vi "AdaptToInputs.vi"(0 "XRef":T14, 1 "Term Types":T11, 2 "State In":T1) -> (14 "Reply":T9, 15 "Fatal Error Out":T8, 16 "State Out":T1)   [LabVIEW 2020, in "Parallel Diagram Block.xnode"]
uses:
  Parallel Diagram Block.xnode
  <vilib>/XNodeSupport/XNodeXNodeRef.ctl
  <vilib>/XNodeSupport/XNodeTermTypeIDPairs.ctl
  <vilib>/XNodeSupport/XNodeTermTypeIDPair.ctl
  <vilib>/XNodeSupport/XNodeType.ctl
  <vilib>/XNodeSupport/XNodeString.ctl
  State.ctl
  Parallel Block/Type Descriptor.ctl
  Parallel Block/Direction.ctl
  Parallel Block/Value Type.ctl
  Parallel Block/Terminal Mode.ctl
  Parallel Block/Terminal Type.ctl
  <vilib>/picture/picture.llb/imagedata.ctl
  <vilib>/XNodeSupport/XNodeStringArray.ctl
  <vilib>/XNodeSupport/XNodeErrorCluster.ctl
  <vilib>/XNodeSupport/NI_XNodeSupport.lvlib
  <vilib>/Utility/Data Type/NI_Data Type.lvlib
  Parallel Block/Parallel Block.lvlib
  Parallel Block/Connection/Connection.lvclass
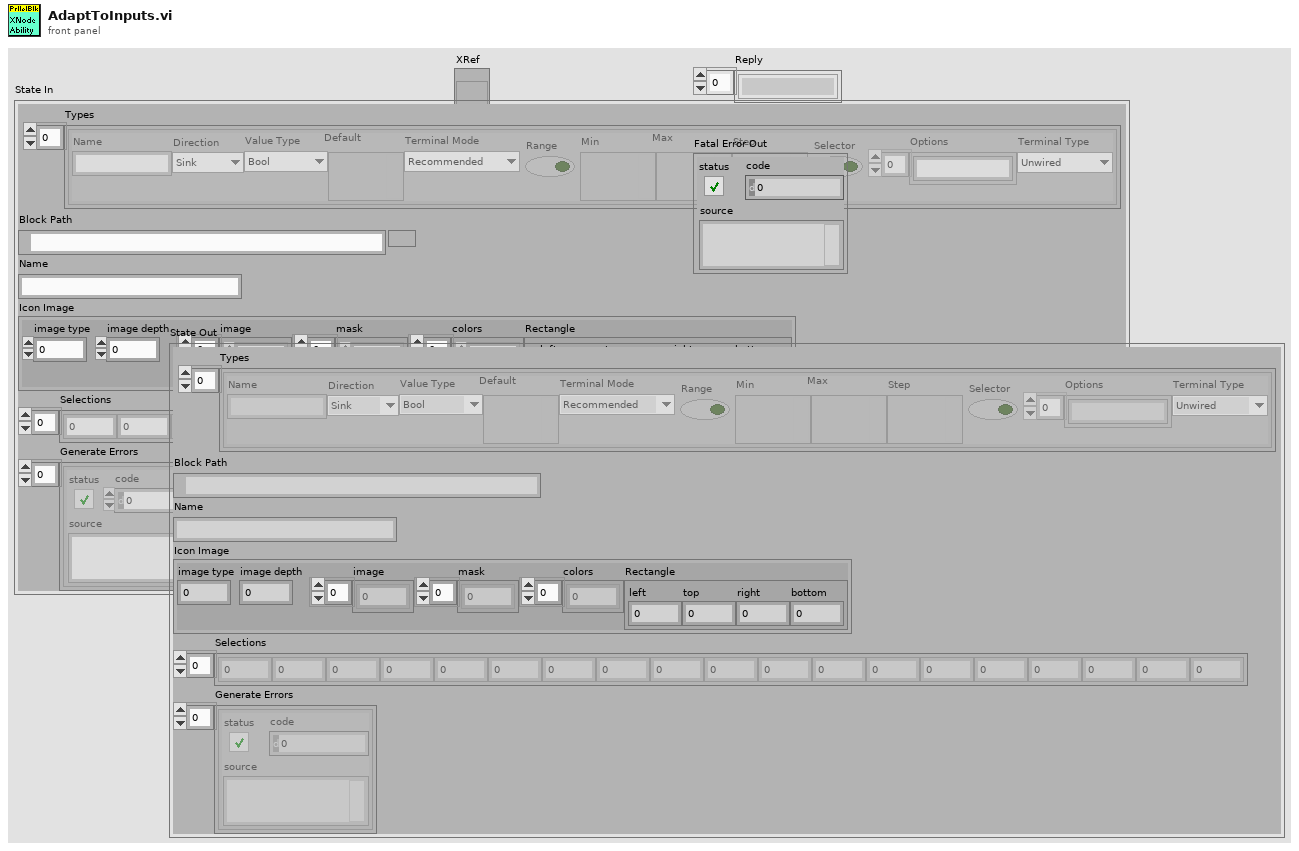
[diagram p1: front panel]
types:
  T1 = typedef "Parallel Diagram Block.xnode/State.ctl" = cluster{"Types":T2[], "Block Path":path, "Name":string, "Icon Image":T7, "Selections":i32[], "Generate Errors":errorcluster[]}
  T2 = typedef "Parallel Block.lvlib/Type Descriptor.ctl" = cluster{"Name":string, "Direction":T3, "Value Type":T4, "Default":variant, "Terminal Mode":T5, "Range":bool, "Min":variant, "Max":variant, "Step":variant, "Selector":bool, "Options":string[], "Terminal Type":T6}
  T3 = typedef "Parallel Block.lvlib/Direction.ctl" = enum16{"Sink", "Source"}
  T4 = typedef "Parallel Block.lvlib/Value Type.ctl" = enum16{"Unknown", "Bool", "U8", "U16", "U32", "U64", "I8", "I16", "I32", "I64", "SGL", "DBL", "CSG", "CDB", "CDBWfm", "String", "DBLWfm"}
  T5 = typedef "Parallel Block.lvlib/Terminal Mode.ctl" = enum16{"Recommended", "Required", "None"}
  T6 = typedef "Parallel Block.lvlib/Terminal Type.ctl" = enum16{"Unwired", "BadType", "Connection", "Value", "Control Ref", "BadRefType"}
  T7 = typedef "imagedata.ctl" = cluster{"image type":i32, "image depth":i32, "image":u8[], "mask":u8[], "colors":u32[], "Rectangle":cluster{"left":i16, "top":i16, "right":i16, "bottom":i16}}
  T8 = typedef "NI_XNodeSupport.lvlib/XNodeErrorCluster.ctl" = errorcluster
  T9 = typedef "NI_XNodeSupport.lvlib/XNodeStringArray.ctl" = T10[]
  T10 = typedef "NI_XNodeSupport.lvlib/XNodeString.ctl" = string
  T11 = typedef "NI_XNodeSupport.lvlib/XNodeTermTypeIDPairs.ctl" = T12[]
  T12 = typedef "NI_XNodeSupport.lvlib/XNodeTermTypeIDPair.ctl" = cluster{"Type":T13, "Id":T10}
  T13 = typedef "NI_XNodeSupport.lvlib/XNodeType.ctl" = variant
  T14 = typedef "NI_XNodeSupport.lvlib/XNodeXNodeRef.ctl" = refnum<vi>
  T15 = typedef "NI_Data Type.lvlib/Data Type.ctl" = enum8{"Invalid Type", "Void", "I8", "I16", "I32", "I64", "U8", "U16", "U32", "U64", "Single Float", "Double Float", "Extended Float", "Single Complex", "Double Complex", "Extended Complex", "Enum U8", "Enum U16", "Enum U32", "Enum U64", "Single Float With Unit", "Double Float With Unit", "Extended Float With Unit", "Single Complex with Unit", "Double Complex with Unit", "Extended Complex with Unit", "Boolean", "String", "Path", "Picture", "Tag", "Array", "Cluster", "Variant", "LV Variant", "Waveform", "Timestamp", "Digital Waveform", "Digital Data", "ExpressData", "Refnum", "External Data", "VI", "Poly VI", "LabVIEW Class Instance", "Fixed Point", "Set Collection", "Map Collection"}
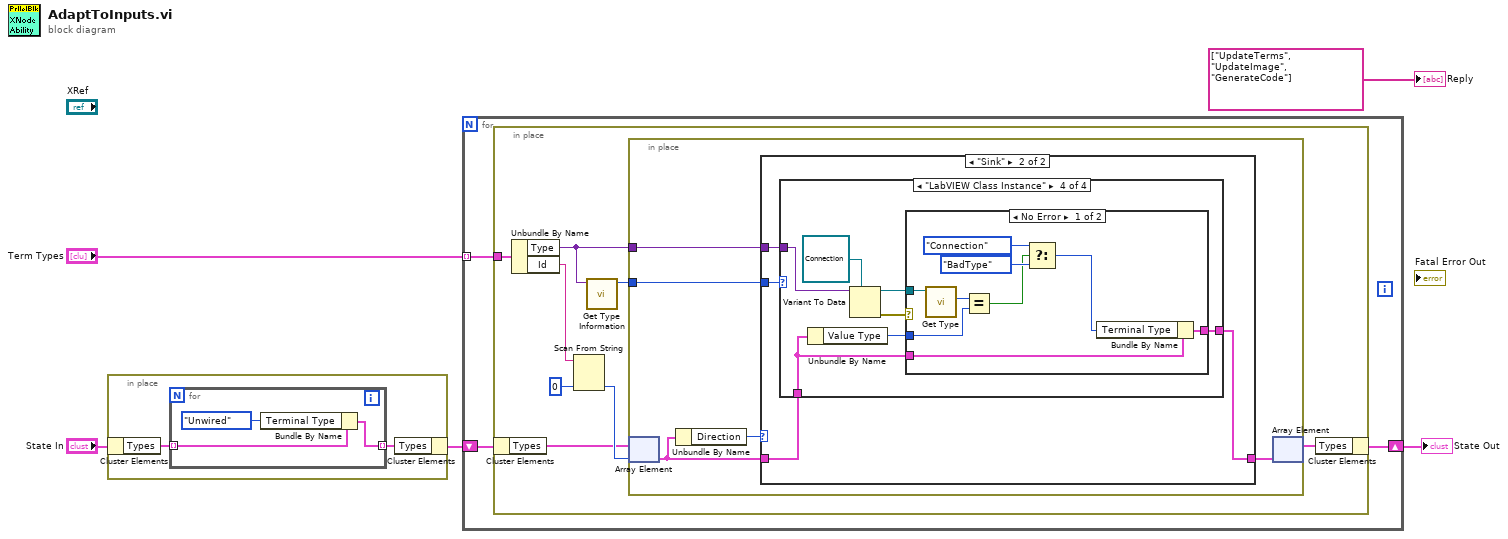
[diagram p0: block diagram]
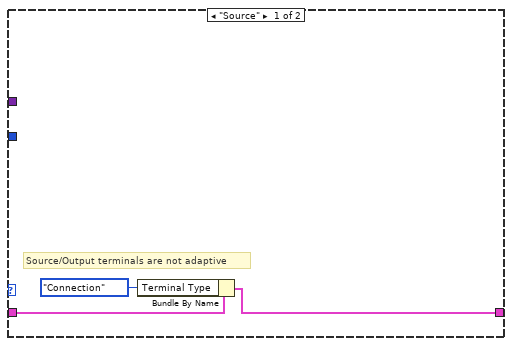
[diagram p2: hidden frame]
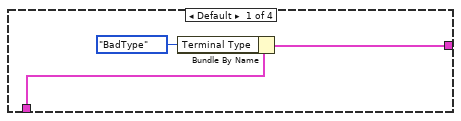
[diagram p3: hidden frame]
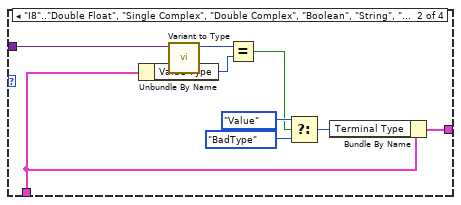
[diagram p4: hidden frame]
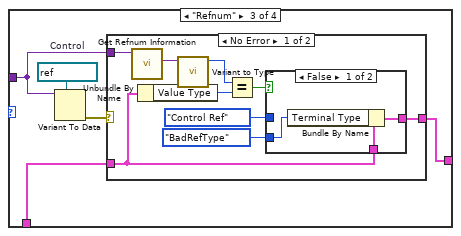
[diagram p5: hidden frame]
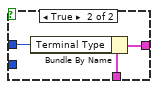
[diagram p6: hidden frame]
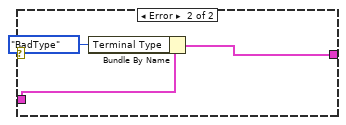
[diagram p7: hidden frame]
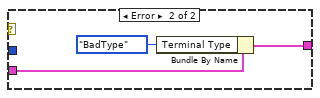
[diagram p8: hidden frame]
diagram:
  n1 = in-place {
    n2 = in-place-cluster #1("State In") -> ("Types"=w7:T2[])
    n3 = for {
      tunnel: w7 -> [w10] mode=indexing
      tunnel: [w8] -> w6 mode=indexing
      n4 = Bundle By Name(cluster=w10, "Terminal Type"=Terminal_Type."Unwired") -> (w8:T2)
    }
    n5 = in-place-cluster #1("Types"=w6) -> (w1:T1)
  }
  n6 = for {
    tunnel: "Term Types" -> [w13] mode=indexing
    shift-right: [w11] -> w3
    shift-left: w1 -> [w12]
    n7 = in-place {
      in-place-border: w13 -> [w21]
      n8 = in-place-cluster #2(w12) -> ("Types"=w14:T2[])
      n9 = Unbundle By Name(w21) -> ("Type"=w17:T13, "Id"=w19:T10)
      n10 = Scan From String(input string=w19, default 1=0) -> (output 1=w16:i32)  [unwired: 3 in, 3 out]
      n11 = call <vilib>:"Get Type Information.vi"("variant"=w17) -> ("type"=w18:T15)  [unwired: 6 in, 4 out]
      n12 = in-place {
        in-place-border: w18 -> [w26]
        in-place-border: w17 -> [w25]
        n13 = in-place-array #3(w14, w16) -> (w23:T2)
        n14 = Unbundle By Name(w23) -> ("Direction"=w22:T3)
        n15 = case shown="\"Sink\"" w22 {
          tunnel: w26 -> [_ w33]
          tunnel: w25 -> [_ w32]
          tunnel: [w28 w31] -> w24
          tunnel: w23 -> [w29 w30]
          frame "Source" {
            # "Source/Output terminals are not adaptive"
            n16 = Bundle By Name(cluster=w29, "Terminal Type"=Terminal_Type."Connection") -> (w28:T2)
          }
          frame "Sink" {
            n17 = case shown="\"LabVIEW Class Instance\"" w33 {
              tunnel: w32 -> [_ w45 w47 w75]
              tunnel: w30 -> [w36 w42 w46 w70]
              tunnel: [w35 w37 w48 w72] -> w31
              frame Default {
                n18 = Bundle By Name(cluster=w36, "Terminal Type"=Terminal_Type."BadType") -> (w35:T2)
              }
              frame "I8".."Double Float", "Single Complex", "Double Complex", "Boolean", "String", "Cluster" {
                n19 = Unbundle By Name(w42) -> ("Value Type"=w44:T4)
                n20 = call "Variant to Type.vi"("Value"=w45) -> ("Value Type"=w43:T4)  [unwired: 10 in]
                n21 = Equal?(x=w43, y=w44) -> (x = y?=w39:bool)
                n22 = Select(t=Terminal_Type."Value" ("Terminal Type"), s=w39, f=Terminal_Type."BadType" ("Terminal Type")) -> (s? t:f=w38:T6)
                n23 = Bundle By Name(cluster=w42, "Terminal Type"=w38) -> (w37:T2)
              }
              frame "Refnum" {
                w50 = refnum<vi> refnum  # Control
                n24 = Variant To Data(type=w50, Variant=w47) -> (error out=w49:errorcluster)  [unwired: 1 in, 1 out]
                n25 = case shown="No Error" w49 {
                  tunnel: w46 -> [w56 w68]
                  tunnel: [w59 w66] -> w48
                  tunnel: w47 -> [w52 _]
                  frame No Error {
                    n26 = call <vilib>:"Get Refnum Information.vi"("variant"=w52) -> ("strict type"=w58:variant)  [unwired: 7 in, 3 out]
                    n27 = Unbundle By Name(w56) -> ("Value Type"=w55:T4)
                    n28 = call "Variant to Type.vi"("Value"=w58) -> ("Value Type"=w57:T4)  [unwired: 10 in]
                    n29 = Equal?(x=w57, y=w55) -> (x = y?=w54:bool)
                    n30 = case shown="False" w54 {
                      tunnel: [w61 w65] -> w59
                      tunnel: w56 -> [w62 w64]
                      tunnel: Terminal_Type."Control Ref" ("Terminal Type") -> [_ w63]
                      tunnel: Terminal_Type."BadRefType" ("Terminal Type") -> [w60 _]
                      frame False {
                        n31 = Bundle By Name(cluster=w62, "Terminal Type"=w60) -> (w61:T2)
                      }
                      frame True {
                        n32 = Bundle By Name(cluster=w64, "Terminal Type"=w63) -> (w65:T2)
                      }
                    }
                  }
                  frame Error {
                    n33 = Bundle By Name(cluster=w68, "Terminal Type"=Terminal_Type."BadType") -> (w66:T2)
                  }
                }
              }
              frame "LabVIEW Class Instance" {
                n34 = Unbundle By Name(w70) -> ("Value Type"=w69:T4)
                n35 = Variant To Data(type=refnum<class "Connection.lvclass"> refnum ("Parallel Block.lvlib:Connection.lvclass"), Variant=w75) -> (data=w71:refnum<class "Connection.lvclass">, error out=w73:errorcluster)  [unwired: 1 in]
                n36 = case shown="No Error" w73 {
                  tunnel: w70 -> [w84 w87]
                  tunnel: [w83 w86] -> w72
                  tunnel: w71 -> [w82 _]
                  tunnel: w69 -> [w81 _]
                  frame No Error {
                    n37 = call-dynamic "Get Type.vi"("Connection in"=w82) -> ("Type"=w80:T4)  [unwired: 8 in, 2 out]
                    n38 = Equal?(x=w80, y=w81) -> (x = y?=w77:bool)
                    n39 = Select(t=Terminal_Type."Connection" ("Terminal Type"), s=w77, f=Terminal_Type."BadType" ("Terminal Type")) -> (s? t:f=w76:T6)
                    n40 = Bundle By Name(cluster=w84, "Terminal Type"=w76) -> (w83:T2)
                  }
                  frame Error {
                    n41 = Bundle By Name(cluster=w87, "Terminal Type"=Terminal_Type."BadType") -> (w86:T2)
                  }
                }
              }
            }
          }
        }
        n42 = in-place-array #3(w24) -> (w15:T2[])  [unwired: 1 out]
      }
      n43 = in-place-cluster #2("Types"=w15) -> (w11:T1)
    }
  }
  "State Out" <- w3
  "Reply" <- T9 ["UpdateTerms", "UpdateImage", "GenerateCode"] ("Reply")
